vi "Step.vi"(0 "State in":refnum<class "State.lvclass">, 1 "Reset":bool, 2 "Stop in":bool, 3 "Start in":bool, 5 "t":u32, 7 "Nt":u32, 9 "C_table":cluster{"C":bool, "NC":u32}[](array[cluster]), 12 "N end step":u32=1) -> (4 "State out":refnum<class "State.lvclass">, 6 "N next":u32, 8 "N curr":u32, 10 "T (ms)":u32)   [LabVIEW 2019, in "Userlib.lvlib" / "State.lvclass"]
uses:
  State.lvclass
  State.lvclass/State.ctl
  Trigers/Triggers.lvlib
  Timer Delay/Timers.lvlib
panel:
  out "Stop out":bool
  out "End":bool
  out "Start out":bool
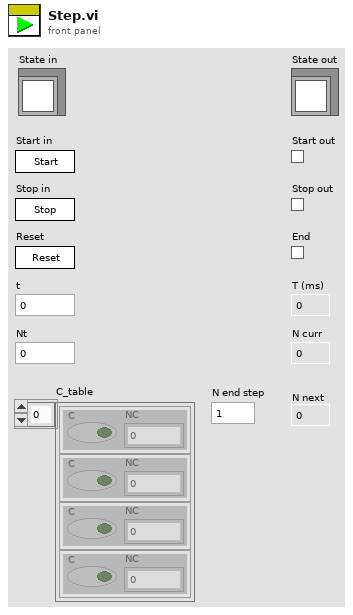
[diagram p1: front panel]
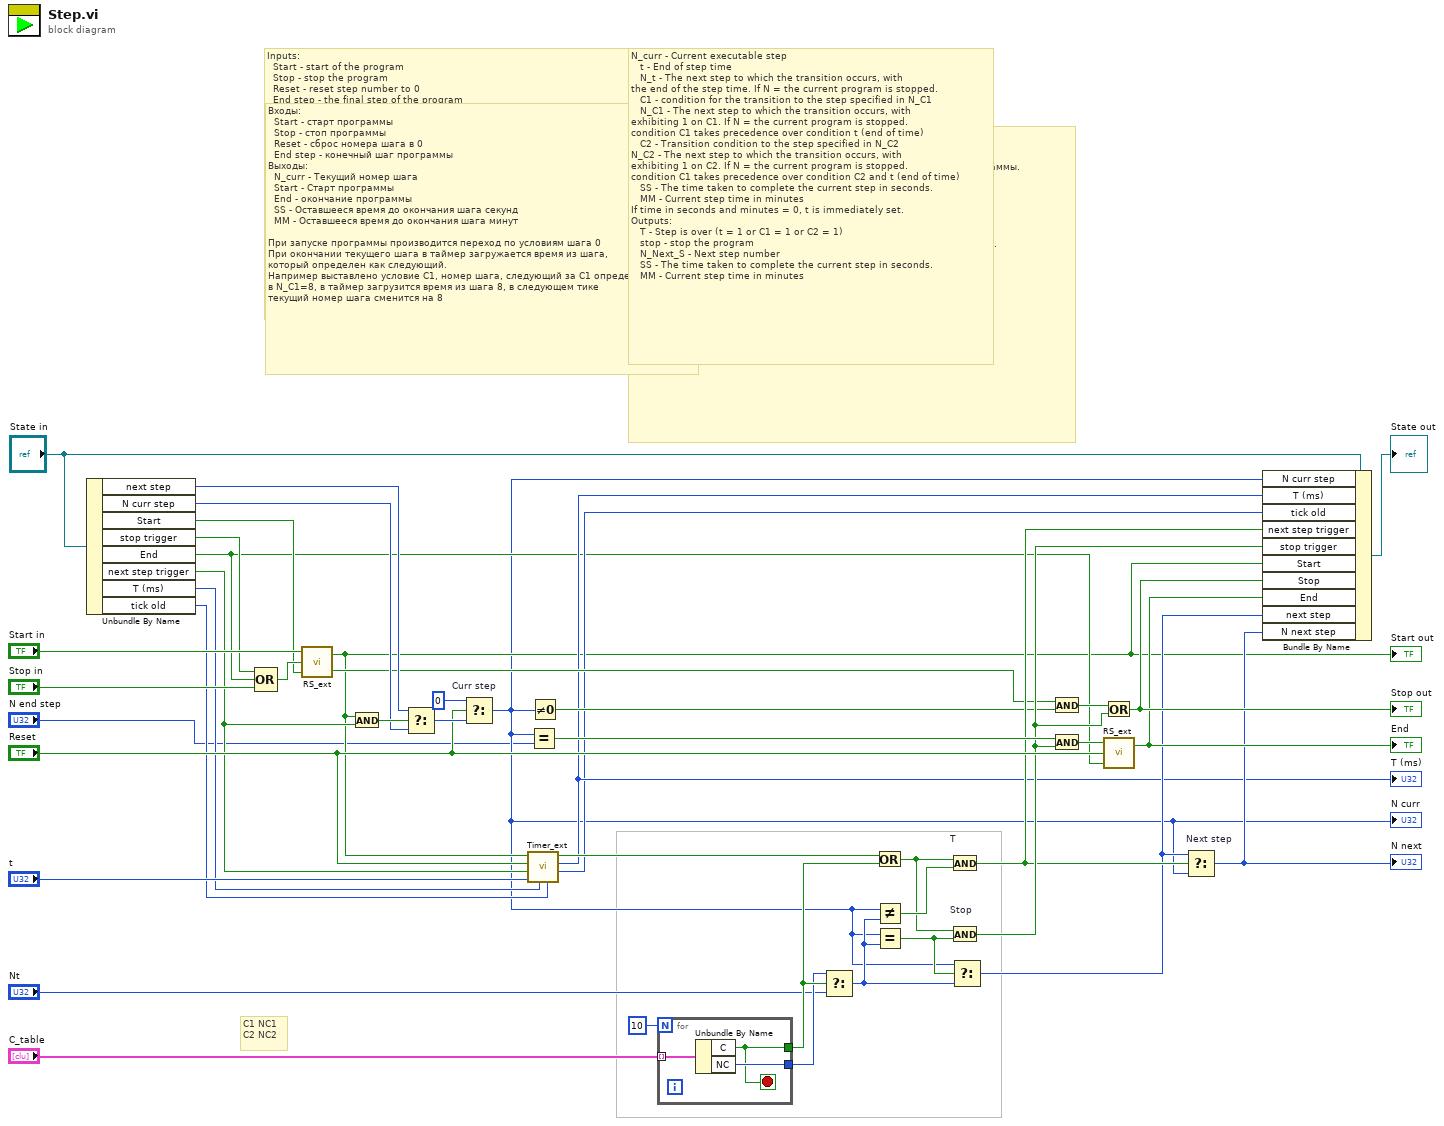
[diagram p0: block diagram]
diagram:
  # "C1 NC1\nC2 NC2"
  # "N_curr - Current executable step\n   t - End of step time\n   N_t - The next step to which the transition occurs, with\nthe end of the step time. If N = the current program is stopped.\n   C1 - condition for the transition to the step specified in N_C1\n   N_C1 - The next step to which the transition occurs, with\nexhibiting 1 on C1. If N = the current program is stopped.\ncondition C1 takes precedence over condition t (end of time)\n   C2 - Transition condition to the step specified in N_C2\nN_C2 - The next step to which the transition occurs, with\nexhibiting 1 on C2. If N = the current program is stopped.\ncondition C1 takes precedence over condition C2 and t (end of time)\n   SS - The time taken to complete the current step in seconds.\n   MM - Current step time in minutes\nIf time in seconds and minutes = 0, t is immediately set.\nOutputs:\n   T - Step is over (t = 1 or C1 = 1 or C2 = 1)\n   stop - stop the program\n   N_Next_S - Next step number\n   SS - The time taken to complete the current step in seconds.\n   MM - Current step time in minutes"
  # "Inputs:\n  Start - start of the program\n  Stop - stop the program\n  Reset - reset step number to 0\n  End step - the final step of the program\nOutputs:\n  N_curr - Current step number\n  Start - Start of the program\n  End - the end of the program\n  SS - Time remaining until the end of the step seconds\n  MM - Time remaining until the end of the step minutes\n\nWhen starting the program, the transition is performed according to the conditions of step 0\nAt the end of the current step, the time from the step is loaded into the timer,\nwhich is defined as the following.\nFor example, condition C1 is set, the step number following C1 is defined\nin N_C1 = 8, the time from step 8 is loaded into the timer, in the next tick\nthe current step number will change to 8"
  # "N_curr - Текущий выполняемый шаг\n  t - Окончание времени шага\n  N_t - Следующий шаг, к которому происходит переход, при\nокончании времени шага. Если N = текущему происходит останов программы.\n  C1 - Условие перехода к шагу, указанному в N_C1\n  N_C1 - Следующий шаг, к которому происходит переход, при\nвыставлении 1 на С1. Если N =текущему происходит останов программы.\nусловие С1 имеет приоритет над условием t (окончание времени)\n  C2 - Условие перехода к шагу, указанному в N_C2\n  N_C2 - Следующий шаг, к которому происходит переход, при\nвыставлении 1 на С2. Если N = текущему происходит останов программы.\nусловие С1 имеет приоритет над условием С2 и t (окончание времени)\n  SS - Время выполнения текущего шага в секундах\n  MM - Время выполнения текущего шага в минутах\nЕсли время в секундах и минутах = 0, сразу выставляется t\nВыходы:\n  T - Шаг окончен (t=1 или C1=1 или С2=1)\n  stop - остановить программу\n  N_Next_S - Номер следующего шага\n  SS - Время выполнения текущего шага в секундах\n  MM - Время выполнения текущего шага в минутах"
  # "Входы:\n  Start - старт программы\n  Stop - стоп программы\n  Reset - сброс номера шага в 0\n  End step - конечный шаг программы\nВыходы:\n  N_curr - Текущий номер шага\n  Start - Старт программы\n  End - окончание программы\n  SS - Оставшееся время до окончания шага секунд\n  MM - Оставшееся время до окончания шага минут\n\nПри запуске программы производится переход по условиям шага 0\nПри окончании текущего шага в таймер загружается время из шага,\nкоторый определен как следующий.\nНапример выставлено условие C1, номер шага, следующий за С1 определен\nв N_C1=8, в таймер загрузится время из шага 8, в следующем тике \nтекущий номер шага сменится на 8"
  n1 = Unbundle By Name("State in") -> ("next step"=w13:u32, "N curr step"=w16:u32, "Start"=w9:bool, "stop trigger"=w17:bool, "End"=w4:bool, "next step trigger"=w10:bool, "T (ms)"=w8:u32, "tick old"=w7:u32)
  n2 = Compound Arithmetic op=OR(w17, w4, "Stop in") -> (w43:bool)
  n3 = call "RS_ext.vi"("Q old"=w9, "R"=w43, "S"="Start in") -> ("~Q"=w11:bool, "Q"=w3:bool)
  "Start out" <- w3
  n4 = And(x=w3, y=w10) -> (x .and. y?=w44:bool)
  n5 = Select(t=w13, s=w44, f=w16) -> (s? t:f=w35:u32)
  n6 = Select "Curr step"(t=u32 0, s="Reset", f=w35) -> (s? t:f=w2:u32)
  "N curr" <- w2
  n7 = call "Timer_ext.vi"("tick old"=w7, "t ms old"=w8, "ms"="t", "Load"=w10, "Reset"="Reset", "Start"=w3) -> ("tick"=w5:u32, "t ms"=w6:u32, "End"=w36:bool)  [unwired: 3 in]
  "T (ms)" <- w6
  n8 = Equal?(x=w2, y="N end step") -> (x = y?=w34:bool)
  n9 = Not Equal To 0?(x=w2) -> (x != 0?=w12:bool)
  n10 = for {
    N: 10 -> [_]
    tunnel: "C_table" -> [w47] mode=indexing
    tunnel: [w46] -> w27
    tunnel: [w45] -> w28
    stop <- w45 stop-if-true
    n11 = Unbundle By Name(w47) -> ("C"=w45:bool, "NC"=w46:u32)
  }
  n12 = Select(t=w27, s=w28, f="Nt") -> (s? t:f=w31:u32)
  n13 = Or(x=w36, y=w28) -> (x .or. y?=w38:bool)
  n14 = Not Equal?(x=w2, y=w31) -> (x != y?=w39:bool)
  n15 = Equal?(x=w2, y=w31) -> (x = y?=w37:bool)
  n16 = And "T"(x=w38, y=w39) -> (x .and. y?=w18:bool)
  n17 = And "Stop"(x=w38, y=w37) -> (x .and. y?=w19:bool)
  n18 = Select(t=w2, s=w37, f=w31) -> (s? t:f=w15:u32)
  n19 = And(x=w11, y=w12) -> (x .and. y?=w33:bool)
  n20 = And(x=w34, y=w19) -> (x .and. y?=w40:bool)
  n21 = Or(x=w33, y=w19) -> (x .or. y?=w21:bool)
  "Stop out" <- w21
  n22 = call "RS_ext.vi"("Q old"=w4, "R"="Reset", "S"=w40) -> ("Q"=w20:bool)  [unwired: 1 out]
  "End" <- w20
  n23 = Select "Next step"(t=w15, s=w18, f=w2) -> (s? t:f=w14:u32)
  "N next" <- w14
  n24 = Bundle By Name(cluster="State in", "N curr step"=w2, "T (ms)"=w6, "tick old"=w5, "next step trigger"=w18, "stop trigger"=w19, "Start"=w3, "Stop"=w21, "End"=w20, "next step"=w15, "N next step"=w14) -> (→"State out":refnum<class "State.lvclass">)
